vi "Load.vi"(8 "error in":errorcluster, 11 "Gantry in":refnum<class "Gantry Class.lvclass">) -> (0 "error out":errorcluster, 3 "SyringeTool out":refnum<class "SyringeTool Class.lvclass">)   [LabVIEW 2011, in "SyringeTool Class.lvclass"]
uses:
  SyringeTool Class.lvclass
  Gantry Class/Gantry Class.lvclass
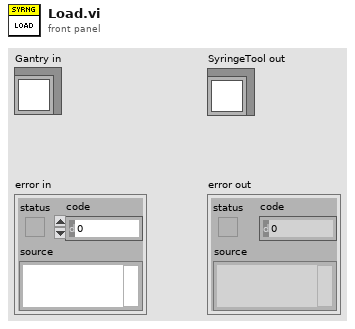
[diagram p1: front panel]
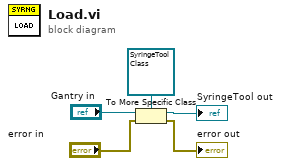
[diagram p0: block diagram]
diagram:
  n1 = To More Specific Class(target class=refnum<class "SyringeTool Class.lvclass"> refnum ("SyringeTool Class in"), reference="Gantry in", error in="error in") -> (specific class reference=→"SyringeTool out":refnum<class "SyringeTool Class.lvclass">, error out=→"error out":errorcluster)
